vi "execution class name.vi"(8 "error in":errorcluster, 11 "Custom Temperature Controller configuration in":refnum<class "Custom Temperature Controller configuration.lvclass">) -> (0 "error out":errorcluster, 2 "class name":string, 3 "Custom Temperature Controller configuration out":refnum<class "Custom Temperature Controller configuration.lvclass">)   [LabVIEW 2021, in "Custom Temperature Controller configuration.lvclass"]
doc: "Provides an interface for determining the module runtime class associated with this module configuration. This class name can then be used to dynamically load or locate the runtime class for initialization purposes."
uses:
  Custom Temperature Controller configuration.lvclass
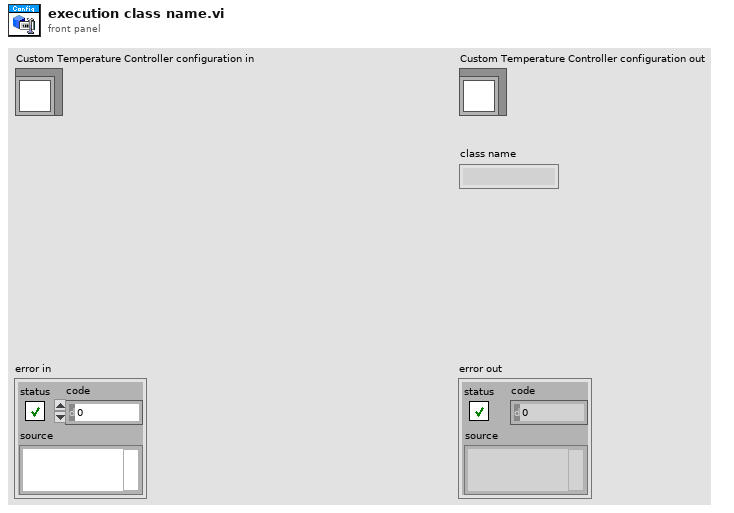
[diagram p1: front panel]
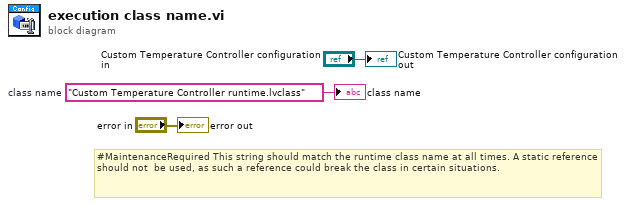
[diagram p0: block diagram]
diagram:
  w1 = "Custom Temperature Controller runtime.lvclass"  # class name
  # "#MaintenanceRequired This string should match the runtime class name at all times. A static reference should not  be used, as such a reference could break the class in certain situations."
  "error out" <- "error in"
  "Custom Temperature Controller configuration out" <- "Custom Temperature Controller configuration in"
  "class name" <- w1
